vi "LFA_GetLastSavedFile.vi"(8 "error in (no error)":errorcluster, 11 "LightField Automation in":refnum<class "LightField Automation.lvclass">) -> (0 "error out":errorcluster, 2 "Data":T1(array[cluster]), 3 "LightField Automation out":refnum<class "LightField Automation.lvclass">)   [LabVIEW 2013, in "LightField Automation.lvclass"]
uses:
  LightField Automation.lvclass
  C:/Program Files/Princeton Instruments/LightField/AddInViews/PrincetonInstruments.LightFieldViewV3.dll
  Program Files/Princeton Instruments/LightField/AddInViews/PrincetonInstruments.LightFieldViewV3.dll
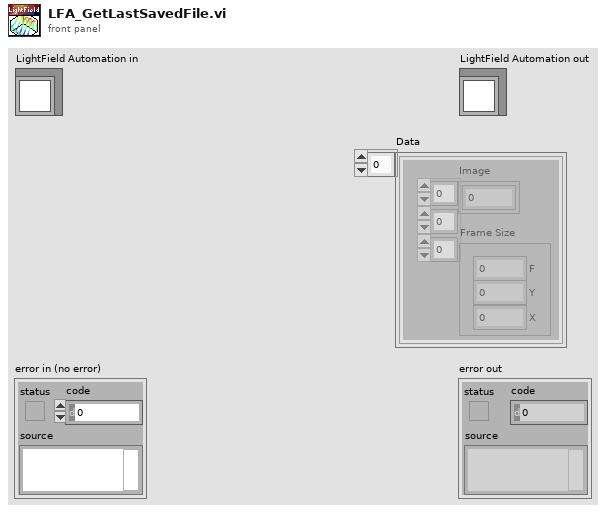
[diagram p1: front panel]
types:
  T1 = cluster{"Image":dbl[][][], "Frame Size":cluster{"F":i32, "Y":i32, "X":i32}}[]
  T2 = cluster{"Image":dbl[][][], "Frame Size":cluster{"F":i32, "Y":i32, "X":i32}}
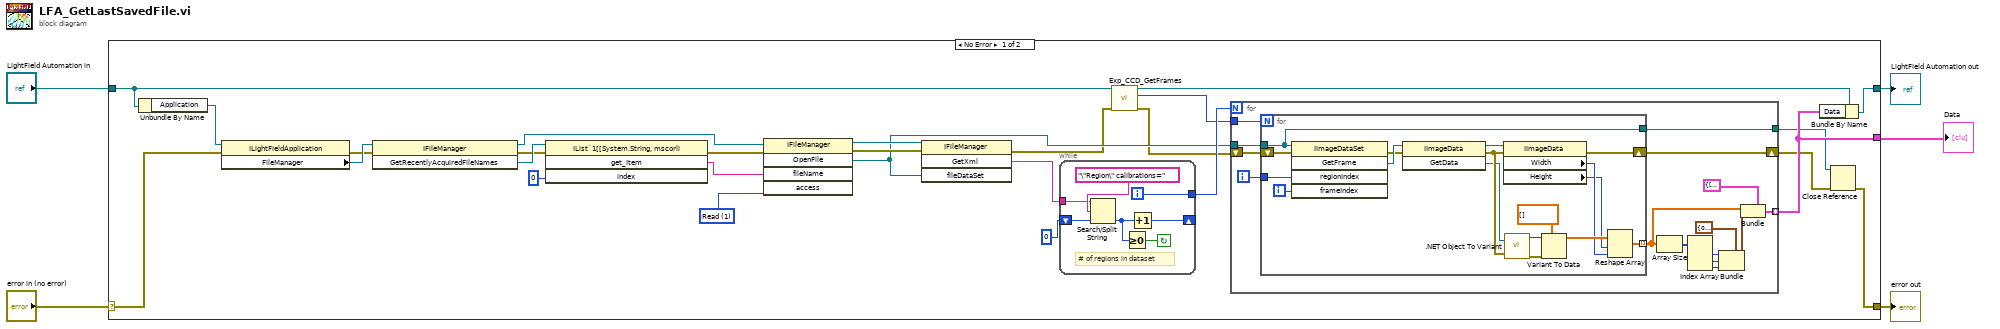
[diagram p0: block diagram]
diagram:
  n1 = case shown="No Error" "error in (no error)" {
    selector: "error in (no error)" -> [w9 w73]
    tunnel: [w7 w73] -> w4
    tunnel: [w13 w72] -> w2
    tunnel: "LightField Automation in" -> [w19 w72]
    tunnel: [w15 _] -> w1
    frame No Error {
      w26 = 1 items=["Read"=1, "Write"=2, "ReadWrite"=3] ("access")
      n2 = Unbundle By Name(w19) -> ("Application"=w12:refnum<k24>)
      n3 = property class="ILightFieldApplication"(reference=w12, error in=w9) -> (error out=w10:errorcluster, "FileManager"=w11:refnum<k24>)  [unwired: 1 out]
      n4 = invoke class="IFileManager" method="GetRecentlyAcquiredFileNames"(reference=w11, error in=w10) -> (reference out=w28:refnum<k24>, error out=w30:errorcluster, "GetRecentlyAcquiredFileNames"=w32:refnum<k24>)  [unwired: 1 in]
      n5 = invoke class="IList`1[[System.String, mscorli" method="get_Item"(reference=w32, error in=w30, "index"=0) -> (error out=w29:errorcluster, "get_Item"=w27:string)  [unwired: 1 in, 2 out]
      n6 = invoke class="IFileManager" method="OpenFile"(reference=w28, error in=w29, "fileName"=w27, "access"=w26) -> (reference out=w25:refnum<k24>, error out=w24:errorcluster, "OpenFile"=w20:refnum<k24>)  [unwired: 1 in, 2 out]
      n7 = invoke class="IFileManager" method="GetXml"(reference=w25, error in=w24, "fileDataSet"=w20) -> (error out=w16:errorcluster, "GetXml"=w23:string)  [unwired: 1 in, 2 out]
      n8 = while {
        tunnel: w23 -> [w69]
        shift-right: [w67] -> _
        shift-left: 0 -> [w68]
        tunnel: [w70] -> w21
        i -> [w70]
        stop <- w65 continue-if-true
        # "# of regions in dataset"
        n9 = Search/Split String(string=w69, search string/char (-)="\"Region\" calibrations=" ("format string"), offset (0)=w68) -> (offset of match=w66:i32)  [unwired: 2 out]
        n10 = Greater Or Equal To 0?(x=w66) -> (x >= 0?=w65:bool)
        n11 = Increment(x=w66) -> (x+1=w67:i32)
      }
      n12 = call "Exp_CCD_GetFrames.vi"("error in (no error)"=w16, "LightField Automation in"=w19) -> ("error out"=w17:errorcluster, "Frames"=w18:i32, "LightField Automation out"=w14:refnum<class "LightField Automation.lvclass">)  [unwired: 7 in]
      n13 = for {
        N: w21 -> [_]
        tunnel: w20 -> [w47]
        shift-right: [w43] -> w8
        shift-left: w17 -> [w46]
        tunnel: w18 -> [w45]
        tunnel: [w40] -> w15 mode=indexing
        tunnel: [w33] -> w6
        i -> [w44]
        n14 = for {
          N: w45 -> [_]
          tunnel: w47 -> [w48]
          tunnel: w44 -> [w62]
          shift-right: [w58] -> w43
          shift-left: w46 -> [w64]
          tunnel: [w49] -> w41 mode=indexing
          tunnel: [w48] -> w33
          i -> [w63]
          n15 = invoke class="IImageDataSet" method="GetFrame"(reference=w48, error in=w64, "regionIndex"=w62, "frameIndex"=w63) -> (error out=w60:errorcluster, "GetFrame"=w61:refnum<k24>)  [unwired: 1 in, 3 out]
          n16 = invoke class="IImageData" method="GetData"(reference=w61, error in=w60) -> (reference out=w59:refnum<k24>, error out=w57:errorcluster, "GetData"=w56:refnum<k24>)  [unwired: 1 in]
          n17 = property class="IImageData"(reference=w59, error in=w57) -> (error out=w58:errorcluster, "Width"=w51:i32, "Height"=w50:i32)  [unwired: 1 out]
          n18 = call <vilib>:".NET Object To Variant.vi"("error in (no error)"=w57, ".NET object"=w56) -> ("error out"=w55:errorcluster, "variant"=w54:variant)
          n19 = Variant To Data(error in=w55, type=dbl[] [], Variant=w54) -> (data=w52:dbl[])  [unwired: 1 out]
          n20 = Reshape Array(w52, w50, w51) -> (w49:dbl[][])
        }
        n21 = Array Size(array=w41) -> (size(s)=w42:i32[])
        n22 = Index Array(array=w42) -> (element #1=w38:i32, element #2=w39:i32, element #3=w37:i32)  [unwired: 3 in]
        n23 = Bundle(cluster=cluster{"F":i32, "Y":i32, "X":i32} {"F"=0, "Y"=0, "X"=0} ("Frame Size"), "F"=w38, "Y"=w39, "X"=w37) -> (w34:cluster{"F":i32, "Y":i32, "X":i32})
        n24 = Bundle(cluster=T2 {"Image"=[], "Frame Size"={"F"=0, "Y"=0, "X"=0}} ("Cluster"), "Image"=w41, "Frame Size"=w34) -> (w40:T2)
      }
      n25 = Bundle By Name(cluster=w14, "Data"=w15) -> (w13:refnum<class "LightField Automation.lvclass">)
      n26 = Close Reference(reference=w6, error in (no error)=w8) -> (error out=w7:errorcluster)
    }
    frame Error {
    }
  }
  "error out" <- w4
  "LightField Automation out" <- w2
  "Data" <- w1
